vi "Comparador.vi"() -> ()   [LabVIEW 2019]
uses:
  <vilib>/Native 3D Graph/xcontrol/3DPC_SurfacePlot.xctl
  <vilib>/Analysis/_algsub.llb/Real Vector Norm.vi
  <vilib>/Utility/file.llb/Read Delimited Spreadsheet (DBL).vi
  <vilib>/Analysis/polynomials.llb/Polynomial Roots (DBL).vi
  <vilib>/Analysis/NI_AALPro.lvlib
  <vilib>/Analysis/NI_AAL_Geometry.lvlib
panel:
  out "chegada":dbl[](array[numeric])
  out "partida":dbl[](array[numeric])
  out "Areas dos triangulos":dbl[](array[numeric])
  out "Primeiro":dbl[](array[numeric])
  out "Ultimo":dbl[](array[numeric])
  out "origem z":dbl
  out "origem y":dbl
  out "origem x":dbl
  out "Roots YZ":cdb[](array[numeric])
  out "Roots XZ":cdb[](array[numeric])
  out "3D Graph 2":refnum<class "Base Datatype.lvclass">[](xcontrol)
  out "Right 2":cluster{"Y":dbl[], "Y":dbl[]}[](graph)
  out "Front 2":cluster{"Y":dbl[], "Y":dbl[]}[](graph)
  out "Top 2":cluster{"Y":dbl[], "Y":dbl[]}[](graph)
  out "Right":cluster{"Y":dbl[], "Y":dbl[]}[](graph)
  out "Front":cluster{"Y":dbl[], "Y":dbl[]}[](graph)
  out "Top":cluster{"Y":dbl[], "Y":dbl[]}[](graph)
  out "3D Graph":refnum<class "Base Datatype.lvclass">[](xcontrol)
  # "Localizaçao da origem"
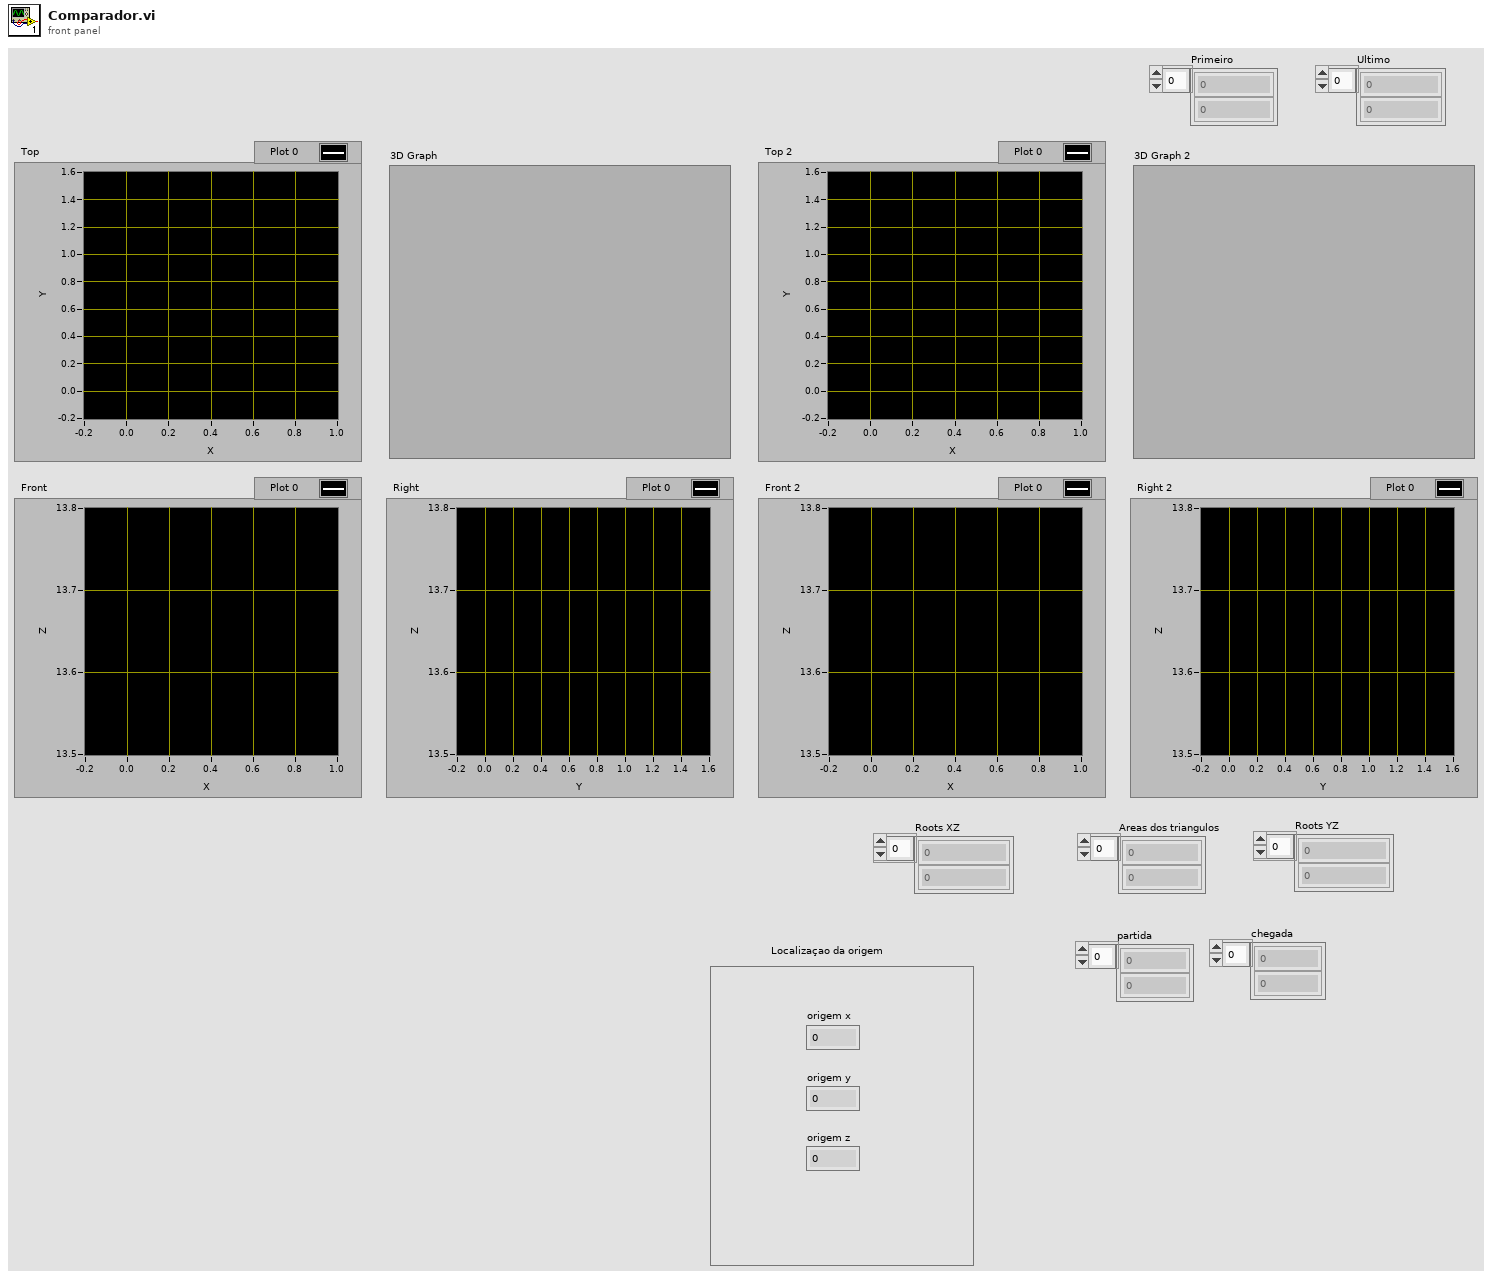
[diagram p1: front panel]
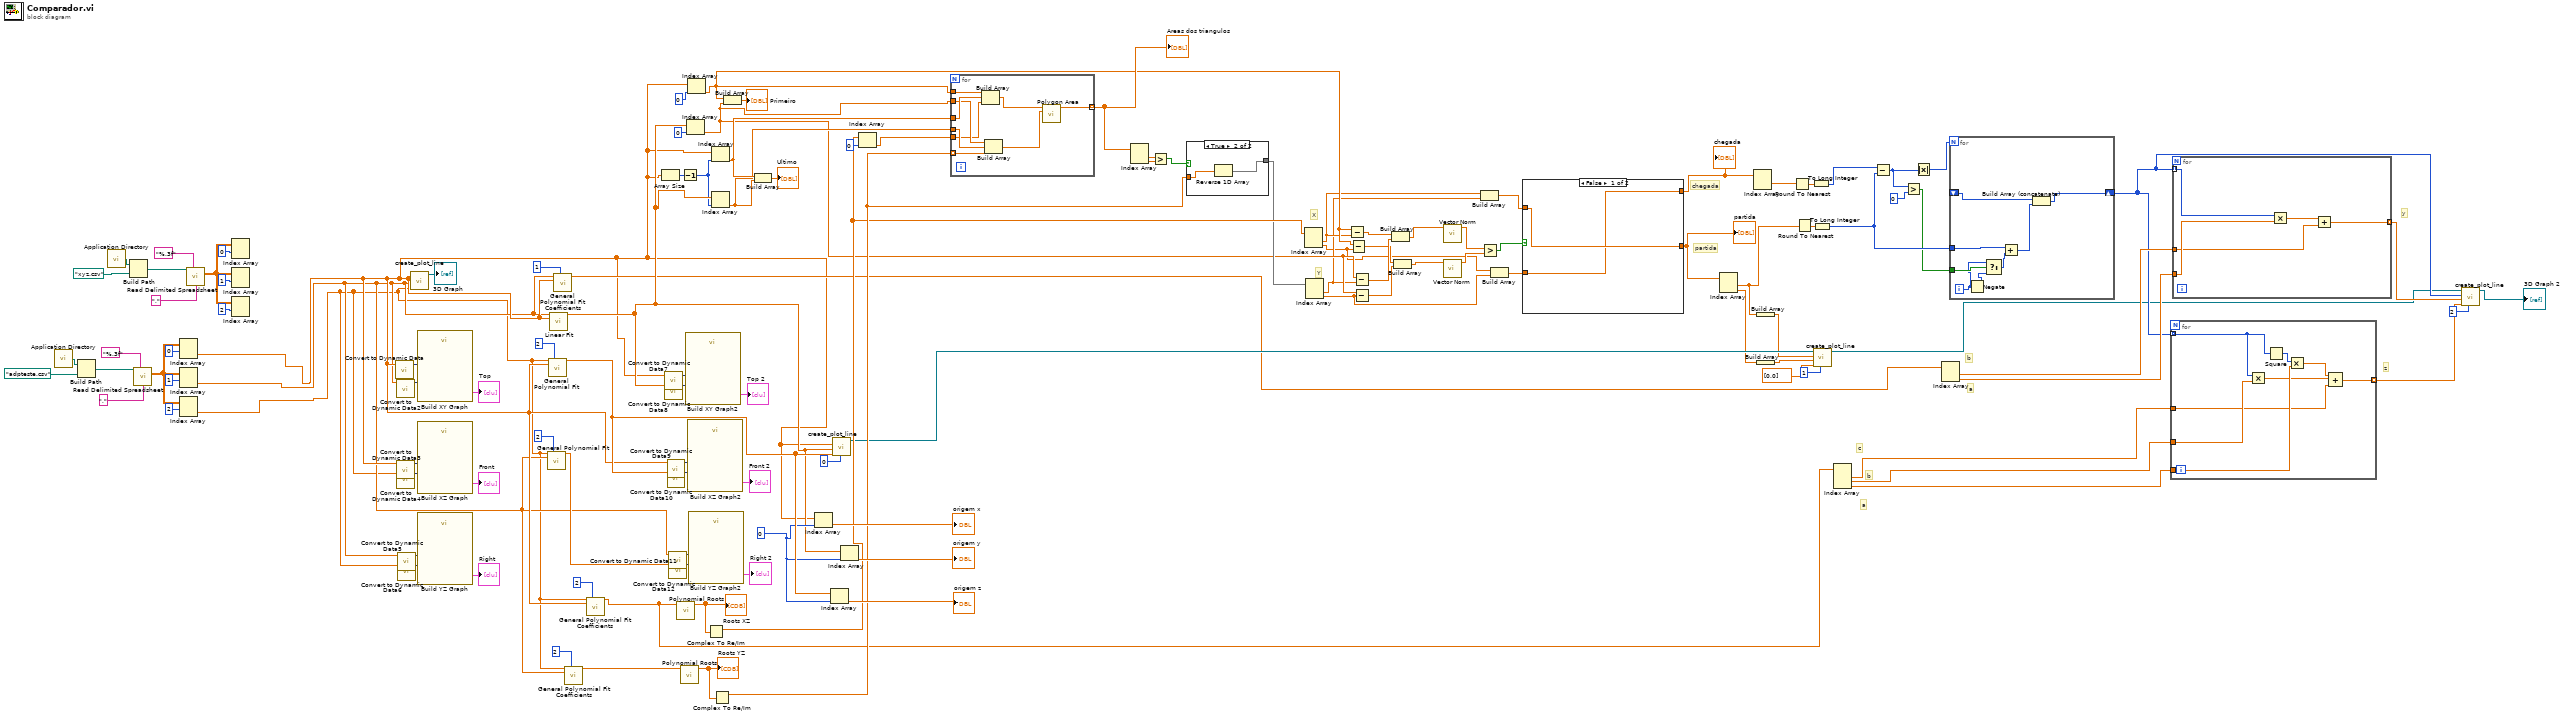
[diagram p0: block diagram]
diagram:
  w74 = 0
  # "y"
  # "z"
  # "b"
  # "a"
  # "c"
  # "b"
  # "a"
  # "partida"
  # "chegada"
  # "Y"
  # "X"
  n1 = call <vilib>:"Application Directory.vi"() -> ("Application Directory"=w85:path)
  n2 = Build Path(base path=w85, name or relative path=path "adpteste.csv" ("file path (dialog if empty)")) -> (appended path=w86:path)
  n3 = call <vilib>:"Application Directory.vi"() -> ("Application Directory"=w119:path)
  n4 = Build Path(base path=w119, name or relative path=path "xyz.csv" ("file path (dialog if empty)")) -> (appended path=w120:path)
  n5 = call-poly <vilib>:"Read Delimited Spreadsheet.vi"("file path (dialog if empty)"=w86, "format (%.3f)"="%.3f", "delimiter (\\t)"="," ("delimiter (\\t)")) -> ("all rows"=w79:dbl[][])  [unwired: 7 in, 5 out]
  n6 = Index Array(array=w79, index (row)=0) -> (element=w3:dbl[])  [unwired: 1 in]
  n7 = Index Array(array=w79, index (row)=1) -> (element=w2:dbl[])  [unwired: 1 in]
  n8 = Index Array(array=w79, index (row)=2) -> (element=w1:dbl[])  [unwired: 1 in]
  n9 = call-poly <vilib>:"Read Delimited Spreadsheet.vi"("file path (dialog if empty)"=w120, "format (%.3f)"="%.3f", "delimiter (\\t)"="," ("delimiter (\\t)")) -> ("all rows"=w112:dbl[][])  [unwired: 7 in, 5 out]
  n10 = Index Array(array=w112, index (row)=0) -> ()  [unwired: 1 in, 1 out]
  n11 = Index Array(array=w112, index (row)=1) -> ()  [unwired: 1 in, 1 out]
  n12 = Index Array(array=w112, index (row)=2) -> ()  [unwired: 1 in, 1 out]
  n13 = call "Convert to Dynamic Data"("Array"=w3) -> ("Dynamic Data Type"=w110:dynamicdata)  [unwired: 3 in]
  n14 = call "Convert to Dynamic Data2"("Array"=w2) -> ("Dynamic Data Type"=w109:dynamicdata)  [unwired: 3 in]
  n15 = call "Convert to Dynamic Data3"("Array"=w3) -> ("Dynamic Data Type"=w106:dynamicdata)  [unwired: 3 in]
  n16 = call "Convert to Dynamic Data4"("Array"=w1) -> ("Dynamic Data Type"=w105:dynamicdata)  [unwired: 3 in]
  n17 = call "Convert to Dynamic Data5"("Array"=w2) -> ("Dynamic Data Type"=w104:dynamicdata)  [unwired: 3 in]
  n18 = call "Convert to Dynamic Data6"("Array"=w1) -> ("Dynamic Data Type"=w103:dynamicdata)  [unwired: 3 in]
  n19 = call <vilib>:"create_plot_line.vi"("z vector"=w1, "y vector"=w2, "x vector"=w3) -> ("plots out"=→"3D Graph":refnum<class "Base Datatype.lvclass">[])  [unwired: 2 in, 6 out]
  n20 = call "Build XY Graph"("Y Input"=w109, "X Input"=w110) -> ("XY Graph"=→"Top":cluster{"X":dbl[], "Y":dbl[]}[])  [unwired: 8 in, 1 out]
  n21 = call "Build XZ Graph"("Y Input"=w105, "X Input"=w106) -> ("XY Graph"=→"Front":cluster{"X":dbl[], "Y":dbl[]}[])  [unwired: 8 in, 1 out]
  n22 = call "Build YZ Graph"("Y Input"=w103, "X Input"=w104) -> ("XY Graph"=→"Right":cluster{"X":dbl[], "Y":dbl[]}[])  [unwired: 8 in, 1 out]
  n23 = call <vilib>:"General Polynomial Fit.vi"("Y"=w1, "polynomial order"=2, "X"=w2) -> ("Best Polynomial Fit"=w91:dbl[])  [unwired: 9 in, 3 out]
  n24 = call <vilib>:"General Polynomial Fit.vi"("Y"=w1, "polynomial order"=2, "X"=w3) -> ("Best Polynomial Fit"=w76:dbl[])  [unwired: 9 in, 3 out]
  n25 = call <vilib>:"Linear Fit.vi"("Y"=w2, "X"=w3) -> ("Best Linear Fit"=w71:dbl[])  [unwired: 9 in, 4 out]
  n26 = call <vilib>:"General Polynomial Fit Coefficients.vi"("Y"=w2, "polynomial order"=1, "X"=w3) -> ("Polynomial Coefficients"=w14:dbl[])  [unwired: 11 in, 1 out]
  n27 = call <vilib>:"General Polynomial Fit Coefficients.vi"("Y"=w1, "polynomial order"=2, "X"=w2) -> ("Polynomial Coefficients"=w88:dbl[])  [unwired: 11 in, 1 out]
  n28 = call <vilib>:"General Polynomial Fit Coefficients.vi"("Y"=w1, "polynomial order"=2, "X"=w3) -> ("Polynomial Coefficients"=w33:dbl[])  [unwired: 11 in, 1 out]
  n29 = Array Size(array=w3) -> (size(s)=w68:i32)
  n30 = call "Convert to Dynamic Data7"("Array"=w3) -> ("Dynamic Data Type"=w101:dynamicdata)  [unwired: 3 in]
  n31 = call "Convert to Dynamic Data8"("Array"=w71) -> ("Dynamic Data Type"=w102:dynamicdata)  [unwired: 3 in]
  n32 = call "Convert to Dynamic Data9"("Array"=w3) -> ("Dynamic Data Type"=w98:dynamicdata)  [unwired: 3 in]
  n33 = call "Convert to Dynamic Data10"("Array"=w76) -> ("Dynamic Data Type"=w99:dynamicdata)  [unwired: 3 in]
  n34 = call "Convert to Dynamic Data11"("Array"=w2) -> ("Dynamic Data Type"=w95:dynamicdata)  [unwired: 3 in]
  n35 = call "Convert to Dynamic Data12"("Array"=w91) -> ("Dynamic Data Type"=w96:dynamicdata)  [unwired: 3 in]
  n36 = call-poly <vilib>:"Polynomial Roots.vi"("P(x)"=w33) -> ("Roots"=w66:cdb[])  [unwired: 9 in, 1 out]
  "Roots XZ" <- w66
  n37 = call-poly <vilib>:"Polynomial Roots.vi"("P(x)"=w88) -> ("Roots"=w65:cdb[])  [unwired: 9 in, 1 out]
  "Roots YZ" <- w65
  n38 = Decrement(x=w68) -> (x-1=w67:i32)
  n39 = call "Build XY Graph2"("Y Input"=w102, "X Input"=w101) -> ("XY Graph"=→"Top 2":cluster{"X":dbl[], "Y":dbl[]}[])  [unwired: 8 in, 1 out]
  n40 = Index Array(array=w71, index=0) -> (element=w52:dbl)
  n41 = Index Array(array=w3, index=0) -> (element=w53:dbl)
  n42 = call "Build XZ Graph2"("Y Input"=w99, "X Input"=w98) -> ("XY Graph"=→"Front 2":cluster{"X":dbl[], "Y":dbl[]}[])  [unwired: 8 in, 1 out]
  n43 = call "Build YZ Graph2"("Y Input"=w96, "X Input"=w95) -> ("XY Graph"=→"Right 2":cluster{"X":dbl[], "Y":dbl[]}[])  [unwired: 8 in, 1 out]
  n44 = Complex To Re/Im(x + iy=w66) -> (x=w55:dbl[])  [unwired: 1 out]
  n45 = Index Array(array=w3, index=w67) -> (element=w64:dbl)
  n46 = Index Array(array=w71, index=w67) -> (element=w63:dbl)
  n47 = Complex To Re/Im(x + iy=w65) -> (x=w56:dbl[])  [unwired: 1 out]
  n48 = Build Array(w53, w52) -> (→"Primeiro":dbl[])
  n49 = Build Array(w64, w63) -> (→"Ultimo":dbl[])
  n50 = Index Array(array=w3, index=w74) -> (element=→"origem x":dbl)
  n51 = Index Array(array=w76, index=w74) -> (element=→"origem z":dbl)
  n52 = call <vilib>:"create_plot_line.vi"("plot ID"=0, "z vector"=w76, "y vector"=w71, "x vector"=w3) -> ("plots out"=w38:refnum<class "Base Datatype.lvclass">[])  [unwired: 1 in, 6 out]
  n53 = Index Array(array=w71, index=w74) -> (element=→"origem y":dbl)
  n54 = Index Array(array=w55, index=0) -> (element=w61:dbl)
  n55 = for {
    tunnel: w56 -> [w126] mode=indexing
    tunnel: w53 -> [w130]
    tunnel: w52 -> [w128]
    tunnel: w64 -> [w129]
    tunnel: w63 -> [w127]
    tunnel: [w123] -> w60 mode=indexing
    tunnel: w61 -> [w122]
    n56 = Build Array(w130, w129, w122) -> (w124:dbl[])
    n57 = Build Array(w128, w127, w126) -> (w125:dbl[])
    n58 = call <vilib>:"Polygon Area.vi"("Y"=w125, "X"=w124) -> ("signed area"=w123:dbl)  [unwired: 8 in, 1 out]
  }
  "Areas dos triangulos" <- w60
  n59 = Index Array(array=w60) -> (element #1=w58:dbl, element #2=w59:dbl)  [unwired: 2 in]
  n60 = Greater?(x=w58, y=w59) -> (0:w57:bool)
  n61 = case shown="True" w57 {
    tunnel: w56 -> [w131 w133]
    tunnel: [w131 w132] -> w54
    frame False {
    }
    frame True {
      n62 = Reverse 1D Array(array=w133) -> (reversed array=w132:dbl[])
    }
  }
  n63 = Index Array(array=w55) -> (element #1=w42:dbl, element #2=w40:dbl)  [unwired: 2 in]
  n64 = Index Array(array=w54) -> (element #1=w41:dbl, element #2=w39:dbl)  [unwired: 2 in]
  n65 = Subtract(x=w53, y=w42) -> (x-y=w51:dbl)
  n66 = Subtract(x=w53, y=w40) -> (x-y=w49:dbl)
  n67 = Subtract(x=w52, y=w41) -> (x-y=w50:dbl)
  n68 = Subtract(x=w52, y=w39) -> (x-y=w48:dbl)
  n69 = Build Array(w51, w50) -> (w44:dbl[])
  n70 = Build Array(w49, w48) -> (w43:dbl[])
  n71 = call-poly <vilib>:"Vector Norm.vi"("Input Vector"=w43) -> ("norm"=w46:dbl)  [unwired: 9 in, 1 out]
  n72 = call-poly <vilib>:"Vector Norm.vi"("Input Vector"=w44) -> ("norm"=w47:dbl)  [unwired: 9 in, 1 out]
  n73 = Build Array(w42, w41) -> (w31:dbl[])
  n74 = Greater?(x=w47, y=w46) -> (0:w45:bool)
  n75 = Build Array(w40, w39) -> (w32:dbl[])
  n76 = case shown="False" w45 {
    tunnel: [w135 w137] -> w30
    tunnel: w32 -> [w134 w137]
    tunnel: w31 -> [w135 w136]
    tunnel: [w134 w136] -> w29
    frame False {
    }
    frame True {
    }
  }
  "partida" <- w30
  "chegada" <- w29
  n77 = Index Array(array=w30) -> (element #1=w27:dbl, element #2=w36:dbl)  [unwired: 2 in]
  n78 = Index Array(array=w29) -> (element #1=w28:dbl)  [unwired: 2 in, 1 out]
  n79 = Build Array(w27) -> (w37:dbl[])
  n80 = Build Array(w36) -> (w35:dbl[])
  n81 = Round To Nearest(number=w28) -> (nearest integer value=w26:dbl)
  n82 = Round To Nearest(number=w27) -> (nearest integer value=w25:dbl)
  n83 = To Long Integer(number=w26) -> (32bit integer=w24:i32)
  n84 = call <vilib>:"create_plot_line.vi"("plot ID"=1, "z vector"=dbl[] [0.0], "y vector"=w35, "x vector"=w37, "plots in"=w38) -> ("plots out"=w8:refnum<class "Base Datatype.lvclass">[])  [unwired: 6 out]
  n85 = To Long Integer(number=w25) -> (32bit integer=w23:i32)
  n86 = Index Array(array=w33) -> (element #1=w16:dbl, element #2=w17:dbl, element #3=w18:dbl)  [unwired: 3 in]
  n87 = Subtract(x=w24, y=w23) -> (x-y=w19:i32)
  n88 = Greater?(x=w19, y=0) -> (0:w20:bool)
  n89 = Absolute Value(x=w19) -> (abs(x)=w22:i32)
  n90 = Index Array(array=w14) -> (element #1=w12:dbl, element #2=w13:dbl)  [unwired: 2 in]
  n91 = for {
    N: w22 -> [_]
    shift-right: [w142] -> w9
    shift-left: _ -> [w145]
    tunnel: w23 -> [w144]
    tunnel: w20 -> [w141]
    i -> [w139]
    n92 = Negate(x=w139) -> (-x=w140:i32)
    n93 = Select(t=w139, s=w141, f=w140) -> (s? t:f=w138:i32)
    n94 = Add(x=w144, y=w138) -> (x+y=w143:i32)
    n95 = Build Array (concatenate)(w145, w143) -> (w142:i32[])
  }
  n96 = for {
    tunnel: w18 -> [w152]
    tunnel: w17 -> [w150]
    tunnel: w16 -> [w147]
    tunnel: w9 -> [w151] mode=indexing
    tunnel: [w146] -> w11 mode=indexing
    n97 = Multiply(x=w151, y=w150) -> (x*y=w148:dbl)
    n98 = Square(x=w151) -> (x^2=w153:i32)
    n99 = Multiply(x=w153, y=w152) -> (x*y=w149:dbl)
    n100 = Compound Arithmetic op=ADD(w149, w148, w147) -> (w146:dbl)
  }
  n101 = for {
    tunnel: w9 -> [w157] mode=indexing
    tunnel: w13 -> [w158]
    tunnel: w12 -> [w156]
    tunnel: [w154] -> w10 mode=indexing
    n102 = Multiply(x=w157, y=w158) -> (x*y=w155:dbl)
    n103 = Add(x=w155, y=w156) -> (x+y=w154:dbl)
  }
  n104 = call <vilib>:"create_plot_line.vi"("plot ID"=2, "z vector"=w11, "y vector"=w10, "x vector"=w9, "plots in"=w8) -> ("plots out"=→"3D Graph 2":refnum<class "Base Datatype.lvclass">[])  [unwired: 6 out]
